vi "Stop All Modules User Event - FGV.vi"(8 "error in":errorcluster, 10 "Action":T1=enum."Get") -> (0 "error out":errorcluster, 3 "Event reference":refnum<user-event>)   [LabVIEW 2018, in "Common.lvlib"]
doc: "Sends a message to all modules to abort and run shutdown code (with cleanup)."
uses:
  Common.lvlib
  ctl/Stop all modules states--enum.ctl
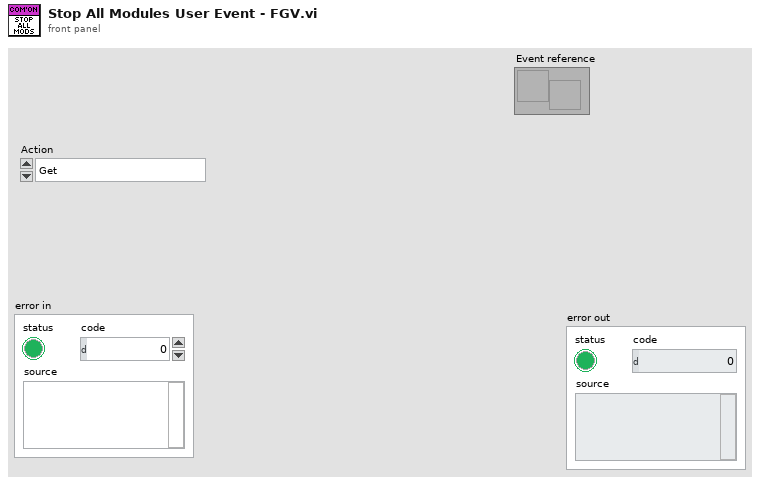
[diagram p1: front panel]
types:
  T1 = typedef "Common.lvlib/Stop all modules states--enum.ctl" = enum16{"Create", "Get", "Send 'Stop all' Message", "Destroy"}
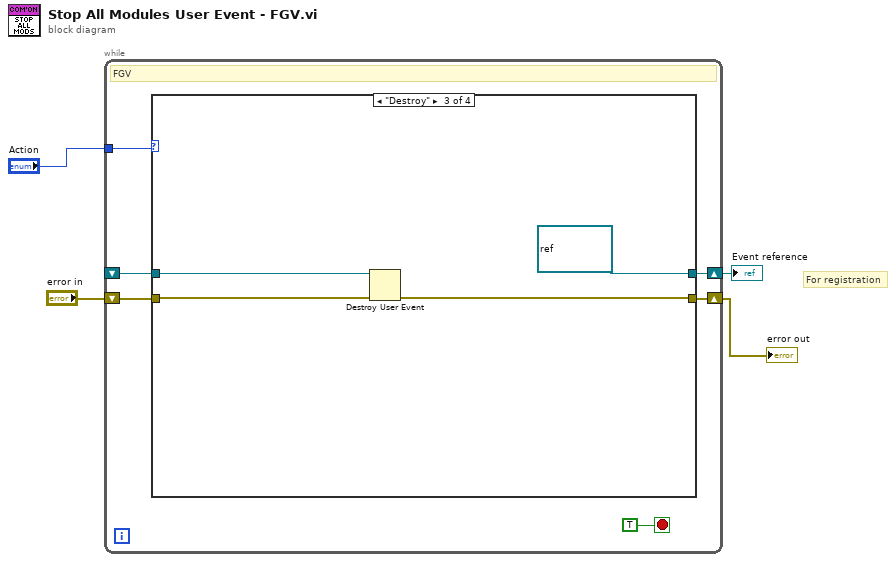
[diagram p0: block diagram]
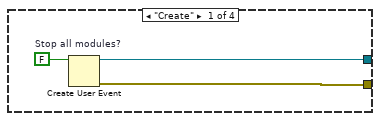
[diagram p2: hidden frame]
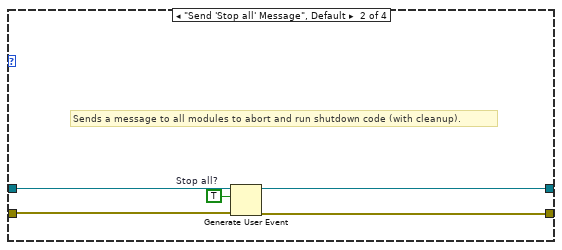
[diagram p3: hidden frame]
diagram:
  # "For registration"
  n1 = while {
    tunnel: "Action" -> [w10]
    shift-right: [w8] -> w3
    shift-left: _ -> [w7]
    shift-right: [w6] -> w2
    shift-left: "error in" -> [w5]
    stop <- TRUE stop-if-true
    # "FGV"
    n2 = case shown="\"Destroy\"" w10 {
      tunnel: [w12 w14 refnum<user-event> refnum ("Stop all modules?") w24] -> w8
      tunnel: w7 -> [_ w18 w21 w24]
      tunnel: [w11 w15 w19 w23] -> w6
      tunnel: w5 -> [_ w16 w20 w23]
      frame "Create" {
        w13 = FALSE  # Stop all modules?
        n3 = Create User Event(user event datatype=w13) -> (user event=w12:refnum<user-event>, error out=w11:errorcluster)  [unwired: 1 in]
      }
      frame "Send 'Stop all' Message", Default {
        w17 = TRUE  # Stop all?
        # "Sends a message to all modules to abort and run shutdown code (with cleanup)."
        n4 = Generate User Event(user event=w18, event data cluster=w17, error in=w16) -> (user event out=w14:refnum<user-event>, error out=w15:errorcluster)  [unwired: 1 in]
      }
      frame "Destroy" {
        n5 = Destroy User Event(user event=w21, error in=w20) -> (error out=w19:errorcluster)
      }
      frame "Get" {
      }
    }
  }
  "Event reference" <- w3
  "error out" <- w2
